vi "Decode Byte.vi"(8 "Step Size (1)":i32=1, 9 "Pixel Offset":i32, 11 "Image In":u8[](array[numeric])) -> (2 "Decoded Byte":u8)   [LabVIEW 2020]
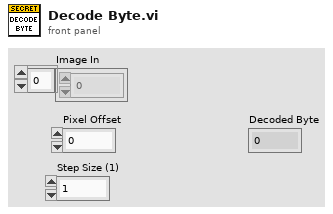
[diagram p1: front panel]
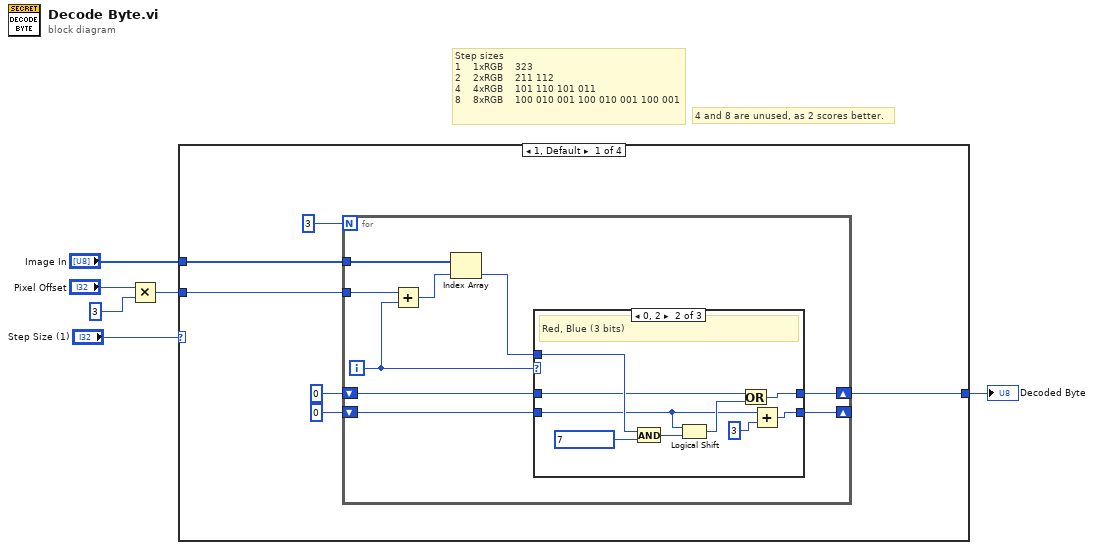
[diagram p0: block diagram]
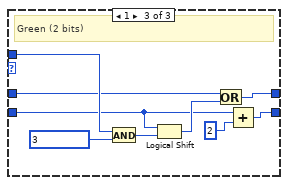
[diagram p3: hidden frame]
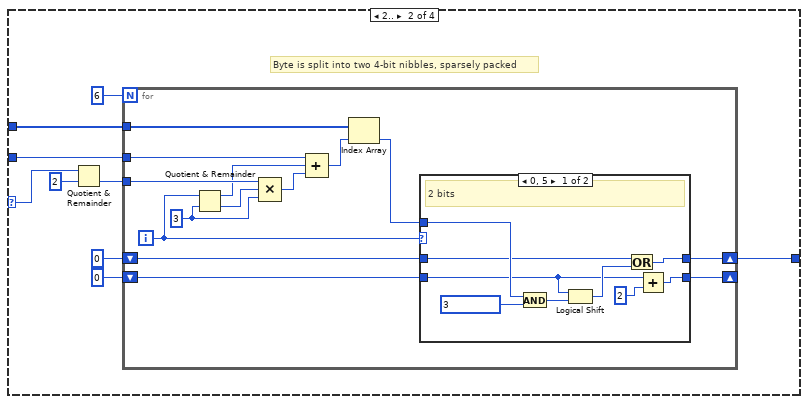
[diagram p4: hidden frame]
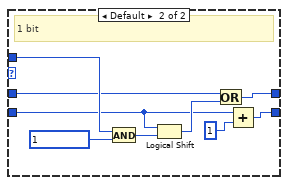
[diagram p5: hidden frame]
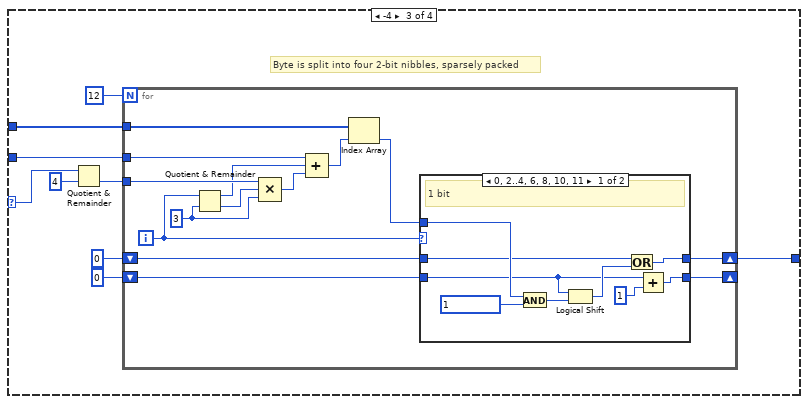
[diagram p6: hidden frame]
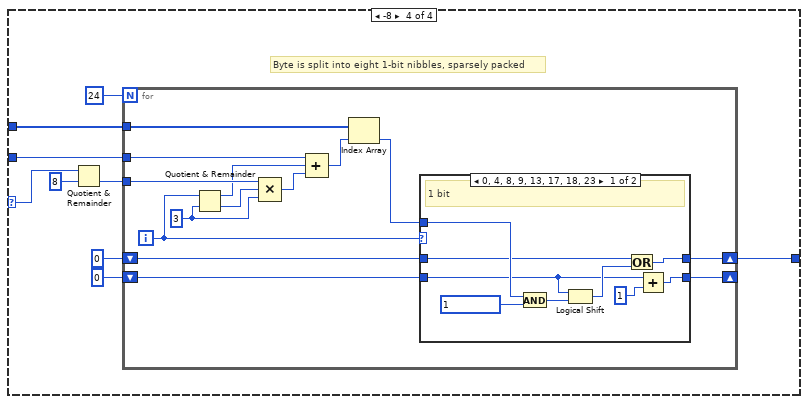
[diagram p8: hidden frame]
diagram:
  # "4 and 8 are unused, as 2 scores better."
  # "Step sizes\n1    1xRGB    323\n2    2xRGB    211 112\n4    4xRGB    101 110 101 011 \n8    8xRGB    100 010 001 100 010 001 100 001"
  n1 = Multiply(x="Pixel Offset", y=3) -> (x*y=w4:i32)
  n2 = case shown="1, Default" "Step Size (1)" {
    selector: "Step Size (1)" -> [_ w43 w84 w118]
    tunnel: w4 -> [w11 w49 w90 w124]
    tunnel: "Image In" -> [w9 w47 w88 w122]
    tunnel: [w8 w46 w87 w121] -> w2
    frame 1, Default {
      n3 = for {
        N: 3 -> [_]
        tunnel: w11 -> [w21]
        shift-right: [w15] -> w8
        shift-left: u8 0 ("y") -> [w19]
        tunnel: w9 -> [w18]
        shift-right: [w13] -> _
        shift-left: i16 0 ("y") -> [w14]
        i -> [w20]
        n4 = Add(x=w21, y=w20) -> (x+y=w17:i32)
        n5 = Index Array(array=w18, index=w17) -> (element=w16:u8)
        n6 = case shown="0, 2" w20 {
          tunnel: w16 -> [_ w30 w39]
          tunnel: w19 -> [w23 w29 w38]
          tunnel: [w23 w27 w36] -> w15
          tunnel: w14 -> [w22 w26 w35]
          tunnel: [w22 w24 w33] -> w13
          frame Default {
          }
          frame 0, 2 {
            # "Red, Blue (3 bits)"
            n7 = And(x=w30, y=u8 7) -> (x .and. y?=w31:u8)
            n8 = Logical Shift(y=w26, x=w31) -> (x << y=w28:u8)
            n9 = Or(x=w29, y=w28) -> (x .or. y?=w27:u8)
            n10 = Add(x=w26, y=i16 3) -> (x+y=w24:i16)
          }
          frame 1 {
            # "Green (2 bits)"
            n11 = And(x=w39, y=u8 3) -> (x .and. y?=w40:u8)
            n12 = Logical Shift(y=w35, x=w40) -> (x << y=w37:u8)
            n13 = Or(x=w38, y=w37) -> (x .or. y?=w36:u8)
            n14 = Add(x=w35, y=i16 2) -> (x+y=w33:i16)
          }
        }
      }
    }
    frame 2.. {
      # "Byte is split into two 4-bit nibbles, sparsely packed"
      n15 = Quotient & Remainder(x=w43, y=2) -> (floor(x/y)=w42:i32)  [unwired: 1 out]
      n16 = for {
        N: 6 -> [_]
        tunnel: w49 -> [w64]
        shift-right: [w59] -> w46
        shift-left: u8 0 ("y") -> [w63]
        tunnel: w47 -> [w62]
        shift-right: [w57] -> _
        shift-left: i16 0 ("y") -> [w58]
        tunnel: w42 -> [w54]
        i -> [w55]
        w53 = 3 ("y")
        n17 = Quotient & Remainder(x=w55, y=w53) -> (x-y*floor(x/y)=w52:i32, floor(x/y)=w56:i32)
        n18 = Compound Arithmetic op=MULTIPLY(w54, w56, w53) -> (w51:i32)
        n19 = Compound Arithmetic op=ADD(w64, w52, w51) -> (w61:i32)
        n20 = Index Array(array=w62, index=w61) -> (element=w60:u8)
        n21 = case shown="0, 5" w55 {
          tunnel: w60 -> [w71 w80]
          tunnel: w63 -> [w70 w79]
          tunnel: [w68 w77] -> w59
          tunnel: w58 -> [w67 w76]
          tunnel: [w65 w74] -> w57
          frame 0, 5 {
            # "2 bits"
            n22 = And(x=w71, y=u8 3) -> (x .and. y?=w72:u8)
            n23 = Logical Shift(y=w67, x=w72) -> (x << y=w69:u8)
            n24 = Or(x=w70, y=w69) -> (x .or. y?=w68:u8)
            n25 = Add(x=w67, y=i16 2) -> (x+y=w65:i16)
          }
          frame Default {
            # "1 bit"
            n26 = And(x=w80, y=u8 1) -> (x .and. y?=w81:u8)
            n27 = Logical Shift(y=w76, x=w81) -> (x << y=w78:u8)
            n28 = Or(x=w79, y=w78) -> (x .or. y?=w77:u8)
            n29 = Add(x=w76, y=i16 1) -> (x+y=w74:i16)
          }
        }
      }
    }
    frame -4 {
      # "Byte is split into four 2-bit nibbles, sparsely packed"
      n30 = Quotient & Remainder(x=w84, y=4) -> (floor(x/y)=w83:i32)  [unwired: 1 out]
      n31 = for {
        N: 12 -> [_]
        tunnel: w90 -> [w105]
        shift-right: [w100] -> w87
        shift-left: u8 0 ("y") -> [w104]
        tunnel: w88 -> [w103]
        shift-right: [w98] -> _
        shift-left: i16 0 ("y") -> [w99]
        tunnel: w83 -> [w95]
        i -> [w96]
        w94 = 3 ("y")
        n32 = Quotient & Remainder(x=w96, y=w94) -> (x-y*floor(x/y)=w93:i32, floor(x/y)=w97:i32)
        n33 = Compound Arithmetic op=MULTIPLY(w95, w97, w94) -> (w92:i32)
        n34 = Compound Arithmetic op=ADD(w105, w93, w92) -> (w102:i32)
        n35 = Index Array(array=w103, index=w102) -> (element=w101:u8)
        n36 = case shown="0, 2..4, 6, 8, 10, 11" w96 {
          tunnel: w101 -> [w112 _]
          tunnel: w104 -> [w111 w116]
          tunnel: [w109 w116] -> w100
          tunnel: w99 -> [w108 w115]
          tunnel: [w106 w115] -> w98
          frame 0, 2..4, 6, 8, 10, 11 {
            # "1 bit"
            n37 = And(x=w112, y=u8 1) -> (x .and. y?=w113:u8)
            n38 = Logical Shift(y=w108, x=w113) -> (x << y=w110:u8)
            n39 = Or(x=w111, y=w110) -> (x .or. y?=w109:u8)
            n40 = Add(x=w108, y=i16 1) -> (x+y=w106:i16)
          }
          frame Default {
            # "0 bits"
          }
        }
      }
    }
    frame -8 {
      # "Byte is split into eight 1-bit nibbles, sparsely packed"
      n41 = Quotient & Remainder(x=w118, y=8) -> (floor(x/y)=w117:i32)  [unwired: 1 out]
      n42 = for {
        N: 24 -> [_]
        tunnel: w124 -> [w139]
        shift-right: [w134] -> w121
        shift-left: u8 0 ("y") -> [w138]
        tunnel: w122 -> [w137]
        shift-right: [w132] -> _
        shift-left: i16 0 ("y") -> [w133]
        tunnel: w117 -> [w129]
        i -> [w130]
        w128 = 3 ("y")
        n43 = Quotient & Remainder(x=w130, y=w128) -> (x-y*floor(x/y)=w127:i32, floor(x/y)=w131:i32)
        n44 = Compound Arithmetic op=MULTIPLY(w129, w131, w128) -> (w126:i32)
        n45 = Compound Arithmetic op=ADD(w139, w127, w126) -> (w136:i32)
        n46 = Index Array(array=w137, index=w136) -> (element=w135:u8)
        n47 = case shown="0, 4, 8, 9, 13, 17, 18, 23" w130 {
          tunnel: w135 -> [w146 _]
          tunnel: w138 -> [w145 w150]
          tunnel: [w143 w150] -> w134
          tunnel: w133 -> [w142 w149]
          tunnel: [w140 w149] -> w132
          frame 0, 4, 8, 9, 13, 17, 18, 23 {
            # "1 bit"
            n48 = And(x=w146, y=u8 1) -> (x .and. y?=w147:u8)
            n49 = Logical Shift(y=w142, x=w147) -> (x << y=w144:u8)
            n50 = Or(x=w145, y=w144) -> (x .or. y?=w143:u8)
            n51 = Add(x=w142, y=i16 1) -> (x+y=w140:i16)
          }
          frame Default {
            # "0 bits"
          }
        }
      }
    }
  }
  "Decoded Byte" <- w2
